vi "Insert Before.vi"(8 "error in (no error)":errorcluster, 11 "Test Configs In":T1) -> (0 "error out":errorcluster, 3 "Test Configs Out":T1)   [LabVIEW 2015]
doc: "Insert either a copied array element or default array element before the active array element."
uses:
  Type Defs/Sequence Parameters Ref.ctl
  Type Defs/Sequence Parameters.ctl
  Type Defs/Target Type.ctl
  Type Defs/Variable Data Type.ctl
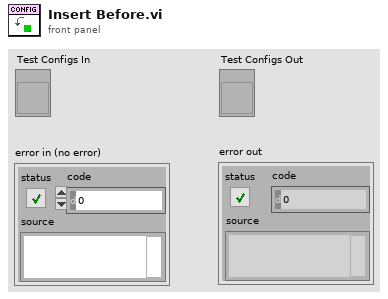
[diagram p1: front panel]
types:
  T1 = typedef "Sequence Parameters Ref.ctl" = refnum<vi>
  T2 = typedef "Sequence Parameters.ctl" = cluster{"Test Name":string, "Target":T3, "Host IP Address":string, "Target IP Address":string, "Shared Variable Host":enum16{"Target", "Host"}, "Shared Variable Writer":enum16{"Target", "Host"}, "Variable Data Type":T4, "# of Variables per Library":u16, "Update Rate (Hz)":dbl, "Read Rate (Hz)":dbl, "Floor":u32, "Ceiling":u32, "Delta":u32}
  T3 = typedef "Target Type.ctl" = enum16{"cRIO-9012", "cRIO-9014", "cRIO-9022", "cRIO-9023", "cRIO-9024", "cRIO-9025", "cRIO-9068", "cRIO-9073", "cRIO-9074", "cRIO-9075", "cRIO-9076", "cRIO-9081", "cRIO-9082", "myRIO-1900", "myRIO-1950", "PXI-8101", "PXI-8115", "PXI-8119", "PXI-8820", "PXIe-8100", "PXIe-8101", "PXIe-8133", "PXIe-8135", "PXIe-8820", "sbRIO-9605", "sbRIO-9606", "sbRIO-9623", "sbRIO-9626", "sbRIO-9633", "sbRIO-9636", "Unlisted (Linux-RT)", "Unlisted (PharLap)", "Unlisted (VxWorks)", "Windows Target"}
  T4 = typedef "Variable Data Type.ctl" = enum16{"U8", "U16", "U32", "U64", "I8", "I16", "I32", "I64", "Single", "Double", "Boolean", "String"}
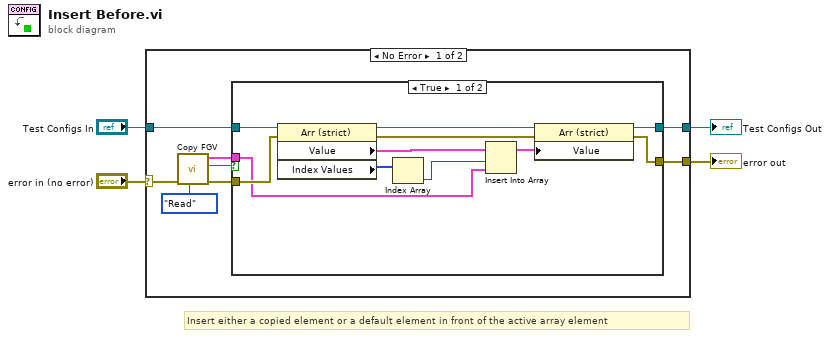
[diagram p0: block diagram]
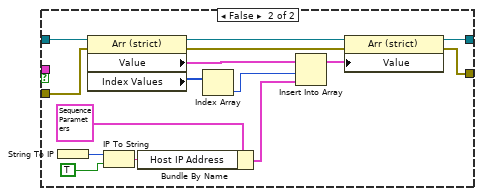
[diagram p2: hidden frame]
diagram:
  # "Insert either a copied element or a default element in front of the active array element"
  n1 = case shown="No Error" "error in (no error)" {
    selector: "error in (no error)" -> [w12 w39]
    tunnel: "Test Configs In" -> [w7 w40]
    tunnel: [w6 w40] -> w1
    tunnel: [w5 w39] -> w2
    frame No Error {
      n2 = call "Copy FGV.vi"("Mode"=enum16{"Enable Copy", "Disable Copy", "Read"}."Read", "error in (no error)"=w12) -> ("error out"=w8:errorcluster, "Copy Enabled? Out"=w10:bool, "Element to Read"=w9:T2)  [unwired: 7 in]
      n3 = case shown="True" w10 {
        tunnel: w9 -> [w19 _]
        tunnel: w8 -> [w22 w37]
        tunnel: w7 -> [w23 w38]
        tunnel: [w15 w31] -> w6
        tunnel: [w14 w30] -> w5
        frame True {
          n4 = property class="Arr (strict)"(reference=w23, error in=w22) -> (reference out=w18:T1, error out=w17:errorcluster, "Value"=w20:T2[], "Index Values"=w21:u32[])
          n5 = Index Array(array=w21) -> (element=w13:u32)  [unwired: 1 in]
          n6 = Insert Into Array(array=w20, index=w13, new element=w19) -> (w16:T2[])
          n7 = property class="Arr (strict)"(reference=w18, error in=w17, "Value"=w16) -> (reference out=w15:T1, error out=w14:errorcluster)
        }
        frame False {
          n8 = String To IP() -> (0:w28:u32)  [unwired: 1 in]
          n9 = property class="Arr (strict)"(reference=w38, error in=w37) -> (reference out=w34:T1, error out=w33:errorcluster, "Value"=w35:T2[], "Index Values"=w36:u32[])
          n10 = IP To String(1:TRUE, 2:w28) -> (0:w26:string)
          n11 = Bundle By Name(cluster=T2 {"Test Name"="Unique Test Name", "Target"=enum."cRIO-9012", "Host IP Address"="0.0.0.0", "Target IP Address"="0.0.0.0", "Shared Variable Host"=enum."Target", "Shared Variable Writer"=enum."Target", "Variable Data Type"=enum."Double", "# of Variables per Library"=500, "Update Rate (Hz)"=1.0, "Read Rate (Hz)"=1.0, "Floor"=500, "Ceiling"=5000, "Delta"=500} ("Test Parameters"), "Host IP Address"=w26) -> (w24:T2)
          n12 = Index Array(array=w36) -> (element=w29:u32)  [unwired: 1 in]
          n13 = Insert Into Array(array=w35, index=w29, new element=w24) -> (w32:T2[])
          n14 = property class="Arr (strict)"(reference=w34, error in=w33, "Value"=w32) -> (reference out=w31:T1, error out=w30:errorcluster)
        }
      }
    }
    frame Error {
    }
  }
  "Test Configs Out" <- w1
  "error out" <- w2
